vi "State_Machine.vi"(8 "error in (no error)":errorcluster caption="entrée d'erreur (pas d'erreur)", 11 "Delay en entrée":refnum<class "Enter_SN.lvclass">) -> (0 "error out":errorcluster caption="sortie d'erreur", 2 "Json_String":string, 3 "Delay en sortie":refnum<class "Enter_SN.lvclass">)   [LabVIEW 2020, in "Library Test.lvlib" / "Enter_SN.lvclass"]
uses:
  Enter_SN.lvclass
  C:/Users/ngarcin/OneDrive - Altyor/Standard TB/Suite TB45/Class/Test/Test (Default)/Test (Default).lvclass
  Popup/Class Popup Operator_Input SN/Class Popup Operator_Input SN.lvclass
  C:/Users/ngarcin/OneDrive - Altyor/Standard TB/Suite TB45/Class/Popup/Class Popup (Main)/Class Popup (Main).lvclass
  Commun VI/TypeDef/Variable Printable.ctl
  JSON API/Variant JSON/Variant JSON.lvlib
  JSON API/Get Polymorphic/JSON GetSet.lvlib
  JSON API/JSON Value/Set from JSON string.vi
  JSON API/JSON Value/JSON Value.lvclass
  Commun VI/Library Commun.lvlib
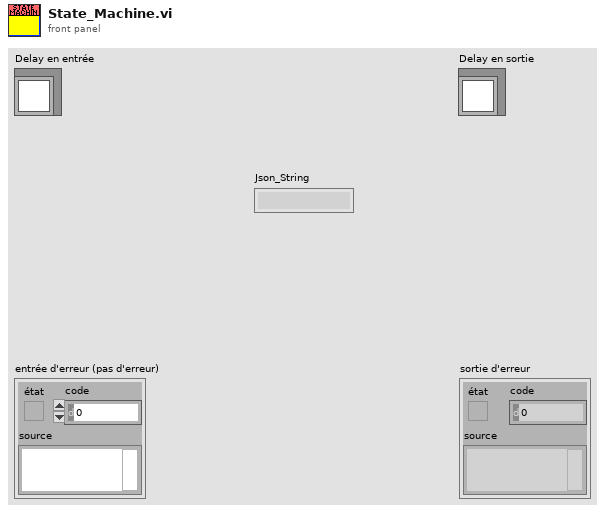
[diagram p1: front panel]
types:
  T1 = enum16{"Get Variable", "Get All Variables", "Set Variable", "Delete Variable", "Delete All Variable"}
  T2 = typedef "Variable Printable.ctl" = string
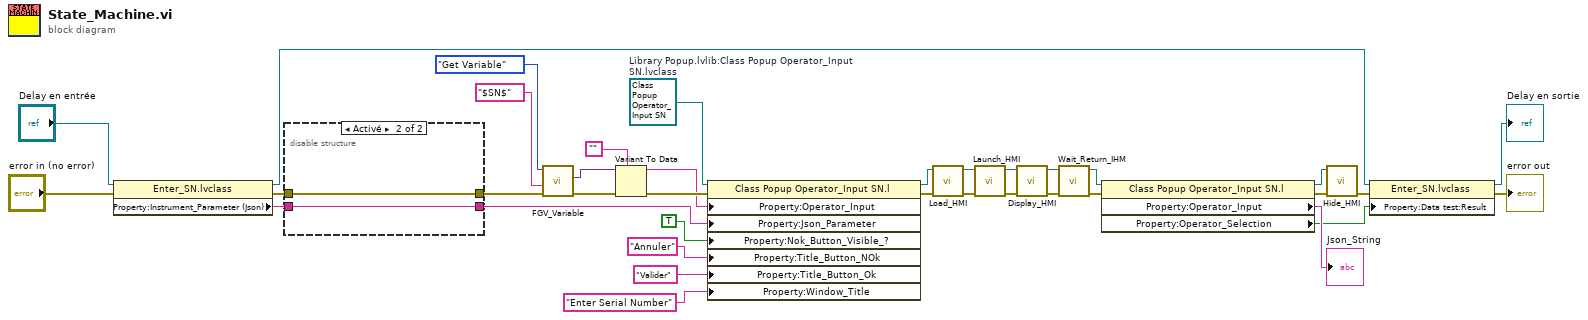
[diagram p0: block diagram]
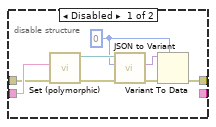
[diagram p2: hidden frame]
diagram:
  w9 = refnum<class "Class Popup Operator_Input SN.lvclass"> refnum  # Library Popup.lvlib:Class Popup Operator_Input SN.lvclass
  n1 = property class="Enter_SN.lvclass"(reference="Delay en entrée", error in="error in (no error)") -> (reference out=w14:refnum<class "Enter_SN.lvclass">, error out=w33:errorcluster, "Property:Instrument_Parameter (Json)"=w35:string)
  n2 = disable-structure shown="Activé" {
    disable-tunnel: w35 -> [w39 w45]
    disable-tunnel: w33 -> [w38 w46]
    disable-tunnel: [w37 w46] -> w3
    disable-tunnel: [_ w45] -> w17
    frame Disabled {
      w40 = u32 0 ("Channel")
      n3 = call-poly "Set (polymorphic).vi"("error in (no error)"=w38, "JSON stream"=w39) -> ("error out"=w42:errorcluster, "JSON Value out"=w44:refnum<class "JSON Value.lvclass">)  [unwired: 7 in, 1 out]
      n4 = call "JSON to Variant.vi"("error in (no error)"=w42, "Variant (Data Type)"=w40, "JSON Value"=w44) -> ("error out"=w43:errorcluster, "Variant out"=w41:variant)  [unwired: 7 in]
      n5 = Variant To Data(error in=w43, type=w40, Variant=w41) -> (error out=w37:errorcluster)  [unwired: 1 out]
    }
    frame Enabled {
    }
  }
  n6 = call "FGV_Variable.vi"("error in (no error)"=w3, "Variable"=T2 "$SN$" ("Variable Printable"), "Function"=T1."Get Variable") -> ("error out"=w7:errorcluster, "Data Out"=w8:variant)  [unwired: 6 in, 1 out]
  n7 = Variant To Data(error in=w7, type="", Variant=w8) -> (data=w1:string, error out=w2:errorcluster)
  n8 = property class="Class Popup Operator_Input SN.l"(reference=w9, error in=w2, "Property:Operator_Input"=w1, "Property:Json_Parameter"=w17, "Property:Nok_Button_Visible_?"=TRUE ("Nok_Button_Visible_?"), "Property:Title_Button_NOk"="Annuler" ("Title_Button_NOk"), "Property:Title_Button_Ok"="Valider" ("Title_Button_Ok"), "Property:Window_Title"="Enter Serial Number" ("Window_Title")) -> (reference out=w26:refnum<class "Class Popup Operator_Input SN.lvclass">, error out=w25:errorcluster)
  n9 = call-dynamic "Load_HMI.vi"("error in (no error)"=w25, "Class Popup (Default) en entrée"=w26) -> ("error out"=w32:errorcluster, "Class Popup (Default) en sortie"=w31:refnum<class "Class Popup Operator_Input SN.lvclass">)  [unwired: 8 in]
  n10 = call-dynamic "Launch_HMI.vi"("error in (no error)"=w32, "Class Popup (Default) en entrée"=w31) -> ("error out"=w30:errorcluster, "Class Popup (Default) en sortie"=w28:refnum<class "Class Popup Operator_Input SN.lvclass">)  [unwired: 8 in]
  n11 = call-dynamic "Display_HMI.vi"("error in (no error)"=w30, "Class Popup (Default) en entrée"=w28) -> ("error out"=w29:errorcluster, "Class Popup (Default) en sortie"=w27:refnum<class "Class Popup Operator_Input SN.lvclass">)  [unwired: 8 in]
  n12 = call-dynamic "Wait_Return_IHM.vi"("error in (no error)"=w29, "Class Popup (Default) en entrée"=w27) -> ("error out"=w21:errorcluster, "Class Popup (Default) en sortie"=w22:refnum<class "Class Popup Operator_Input SN.lvclass">)  [unwired: 8 in]
  n13 = property class="Class Popup Operator_Input SN.l"(reference=w22, error in=w21) -> (reference out=w16:refnum<class "Class Popup Operator_Input SN.lvclass">, error out=w15:errorcluster, "Property:Operator_Input"=→"Json_String":string, "Property:Operator_Selection"=w12:bool)
  n14 = call-dynamic "Hide_HMI.vi"("error in (no error)"=w15, "Class Popup (Default) en entrée"=w16) -> ("error out"=w13:errorcluster)  [unwired: 8 in, 1 out]
  n15 = property class="Enter_SN.lvclass"(reference=w14, error in=w13, "Property:Data test:Result"=w12) -> (reference out=→"Delay en sortie":refnum<class "Enter_SN.lvclass">, error out=→"error out":errorcluster)
